vi "Format Test Filename.vi"(1 "Parameter Table In":string[](array[string]), 2 "start path":path) -> (0 "Full Path":path)   [LabVIEW 2018]
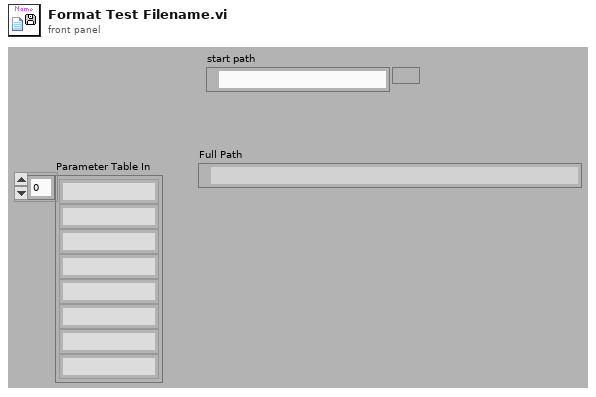
[diagram p1: front panel]
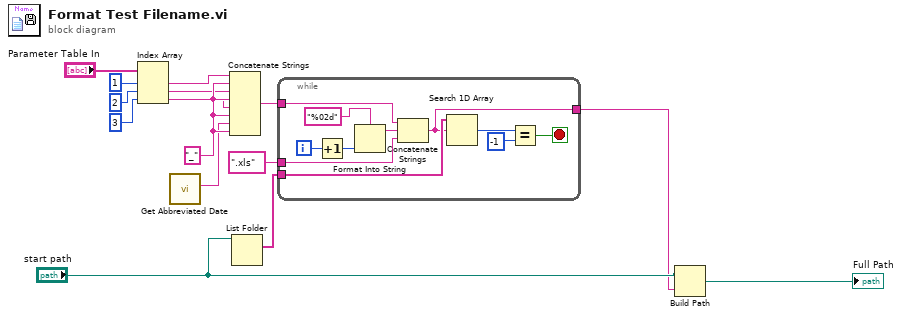
[diagram p0: block diagram]
diagram:
  w14 = "_" ("string")
  n1 = Index Array(array="Parameter Table In", index #1=1 ("index"), index #2=2 ("index"), index #3=3 ("index")) -> (element #1=w6:string, element #2=w8:string, element #3=w10:string)
  n2 = call "Get Abbreviated Date.vi"() -> ("Abrreviated Data"=w11:string)  [unwired: 11 in]
  n3 = Concatenate Strings(w6, w14, w8, w14, w10, w14, w11, w14) -> (w15:string)
  n4 = List Folder(path="start path") -> (filenames=w12:string[])  [unwired: 3 in, 3 out]
  n5 = while {
    tunnel: w12 -> [w26]
    tunnel: ".xls" ("string") -> [w22]
    tunnel: [w18] -> w2
    tunnel: w15 -> [w17]
    i -> [w21]
    stop <- w23 stop-if-true
    n6 = Increment(x=w21) -> (x+1=w16:i32)
    n7 = Format Into String(format string="%02d", w16) -> (resulting string=w20:string)  [unwired: 2 in, 1 out]
    n8 = Concatenate Strings(w17, w20, w22) -> (w18:string)
    n9 = Search 1D Array(1D array=w26, element=w18) -> (index of element=w25:i32)  [unwired: 1 in]
    n10 = Equal?(x=w25, y=-1) -> (x = y?=w23:bool)
  }
  n11 = Build Path(base path="start path", name or relative path=w2) -> (appended path=→"Full Path":path)
